vi "FromRepo.vi"(8 "error in":errorcluster, 9 "from repo cluster":T2, 10 "repository in":refnum<class "NISE_CEF_Repository.lvclass">, 11 "engine in":refnum<class "Engine Parent Editor Node.lvclass">) -> (0 "error out":errorcluster, 2 "repository out":refnum<class "NISE_CEF_Repository.lvclass">, 3 "node":T1)   [LabVIEW 2013, in "PL Framework Configuration Tool.lvlib" / "Engine Parent Editor Node.lvclass"]
doc: "Grabs information from the Repo and stores it in the nodes."
uses:
  Engine Parent Editor Node.lvclass
  <vilib>/CEF_TreeControl/Repository/NISE_CEF_Repository.lvclass
  <vilib>/CEF_TreeControl/Node/FromRepoCluster.ctl
  <vilib>/CEF_TreeControl/Node/NodeRef.ctl
  <vilib>/CEF_TreeControl/Node/NISE_CEF_Node.lvclass
  Framework Configuration Classes/platypus configuration/engines cluster.ctl
  <vilib>/NI/Module Execution Interface/Engine Configuration/engine configuration.lvclass
  <vilib>/NI/Tag Bus Module Framework/module configuration/TBM module configuration.lvclass
  EngineTags/EngineTags.lvclass
  Engine Mappings/Engine Mappings.lvclass
  TBM Configuration Node/TBM Configuration Node.lvclass
  <vilib>/NI/Tag Bus Module Framework/root configuration/TBM configuration.lvclass/TBM configuration.ctl
  Framework Configuration Classes/class cache/class type.ctl
  <vilib>/NI/Tag Bus Module Framework/root configuration/create GUID.vi
  <vilib>/NI/Tag Bus Module Framework/root configuration/read metadata property.vi
  Framework Configuration Classes/class cache/PL_class cache.lvlib
  Framework Configuration Classes/platypus configuration/PLConfigurationSerializer.lvlib
  <vilib>/NI/Tag Bus Module Framework/root configuration/TBM configuration.lvclass
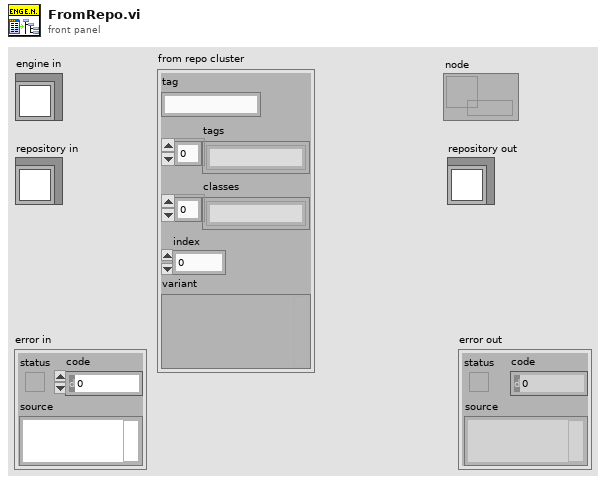
[diagram p1: front panel]
types:
  T1 = typedef "NISE_CEF_Node.lvclass/NodeRef.ctl" = refnum<data-value>
  T2 = typedef "NISE_CEF_Node.lvclass/FromRepoCluster.ctl" = cluster{"tag":string, "tags":string[], "classes":string[], "index":i32, "variant":variant}
  T3 = typedef "PLConfigurationSerializer.lvlib/engines cluster.ctl" = cluster{"engine configuration":refnum<class "engine configuration.lvclass">, "modules":refnum<class "TBM module configuration.lvclass">[]}
  T4 = typedef "PL_class cache.lvlib/class type.ctl" = enum16{"unused", "other pl", "system", "target", "engine", "module"}
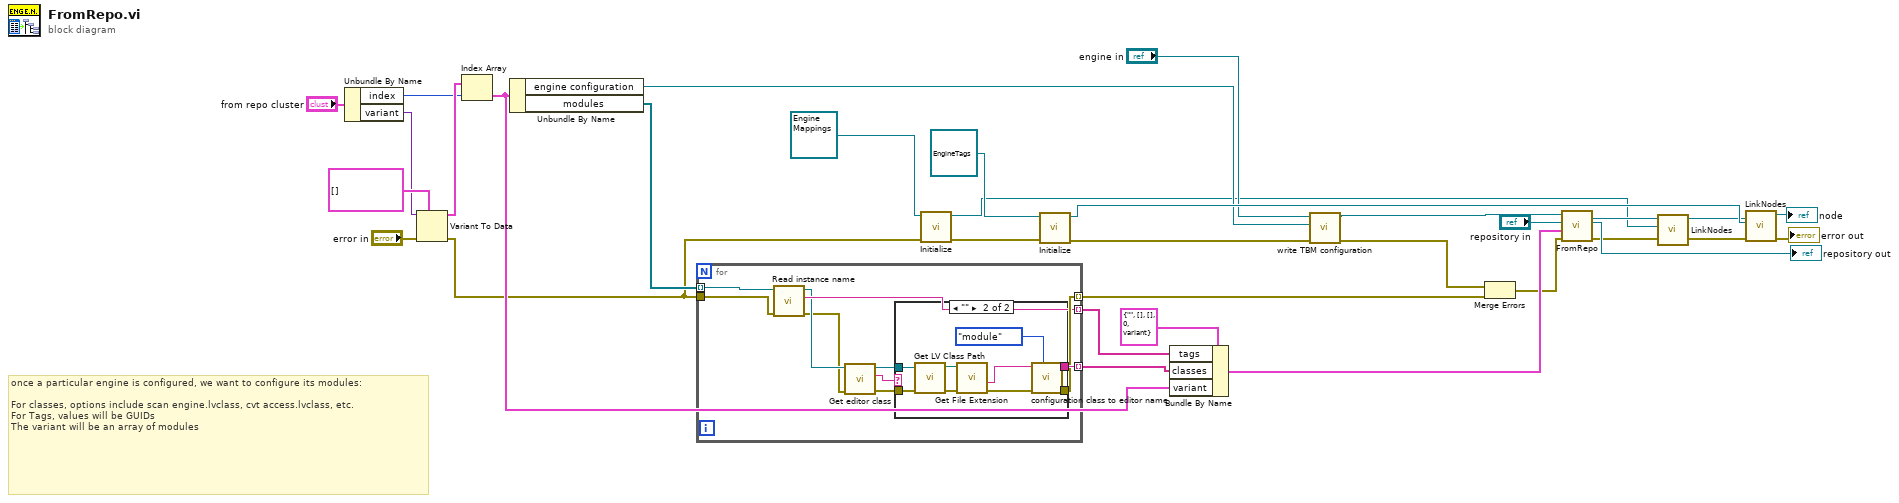
[diagram p0: block diagram]
diagram:
  # "once a particular engine is configured, we want to configure its modules:\n\nFor classes, options include scan engine.lvclass, cvt access.lvclass, etc.\nFor Tags, values will be GUIDs\nThe variant will be an array of modules"
  n1 = Unbundle By Name("from repo cluster") -> ("index"=w31:i32, "variant"=w30:variant)
  n2 = Variant To Data(error in="error in", type=T3[] [], Variant=w30) -> (data=w32:T3[], error out=w1:errorcluster)
  n3 = Index Array(array=w32, index=w31) -> (element=w14:T3)
  n4 = Unbundle By Name(w14) -> ("engine configuration"=w12:refnum<class "engine configuration.lvclass">, "modules"=w15:refnum<class "TBM module configuration.lvclass">[])
  n5 = for {
    tunnel: w15 -> [w43] mode=indexing
    tunnel: [w39] -> w28 mode=indexing
    tunnel: [w42] -> w27 mode=indexing
    tunnel: w1 -> [w40]
    tunnel: [w41] -> w18 mode=indexing
    n6 = call <vilib>:"Read instance name.vi"("error in"=w40, "configuration in"=w43) -> ("error out"=w37:errorcluster, "instance id"=w39:string, "configuration out"=w38:refnum<class "TBM module configuration.lvclass">)  [unwired: 7 in]
    n7 = call "Get editor class.vi"("error in"=w37, "configuration in"=w38) -> ("error out"=w35:errorcluster, "editor class"=w34:string, "configuration out"=w36:refnum<class "TBM module configuration.lvclass">)  [unwired: 7 in]
    n8 = case shown="\"\"" w34 {
      selector: w34 -> [w44 _]
      tunnel: [w44 w54] -> w42
      tunnel: [w45 w52] -> w41
      tunnel: w36 -> [_ w50]
      tunnel: w35 -> [w45 w46]
      frame Default {
      }
      frame "" {
        n9 = call <vilib>:"Get LV Class Path.vi"("error in (no error)"=w46, "object"=w50) -> ("error out"=w51:errorcluster, "class path"=w49:path)  [unwired: 8 in]
        n10 = call <vilib>:"Get File Extension.vi"("error in (no error)"=w51, "file"=w49) -> ("error out"=w47:errorcluster, "filename without extension"=w48:string)  [unwired: 6 in, 2 out]
        n11 = call "configuration class to editor name.vi"("class type"=class_type."module", "error in"=w47, "configuration class name"=w48) -> ("error out"=w52:errorcluster, "editor node class name"=w54:string)  [unwired: 7 in]
      }
    }
  }
  n12 = call-dynamic "Initialize.vi"("error in"=w1, "node in"=refnum<class "Engine Mappings.lvclass"> refnum ("PL Framework Configuration Tool.lvlib:Engine Mapping Viewer")) -> ("error out"=w4:errorcluster, "data value reference"=w2:T1)  [unwired: 7 in, 1 out]
  n13 = call-dynamic "Initialize.vi"("error in"=w4, "node in"=refnum<class "EngineTags.lvclass"> refnum ("EngineTags.lvclass")) -> ("error out"=w11:errorcluster, "data value reference"=w26:T1)  [unwired: 7 in, 1 out]
  n14 = Bundle By Name(cluster=T2 {"tag"="", "tags"=[], "classes"=[], "index"=0, "variant"=variant} ("from repo cluster"), "tags"=w28, "classes"=w27, "variant"=w14) -> (w25:T2)
  n15 = call-dynamic "write TBM configuration.vi"("error in"=w11, "configuration"=w12, "TBM Configuration Node in"="engine in") -> ("error out"=w10:errorcluster, "TBM Configuration Node out"=w9:refnum<class "Engine Parent Editor Node.lvclass">)  [unwired: 7 in]
  n16 = Merge Errors(w10, w18) -> (w17:errorcluster)
  n17 = call-parent "FromRepo.vi"("error in"=w17, "from repo cluster"=w25, "repository in"="repository in", "node in"=w9) -> ("error out"=w8:errorcluster, "repository out"=→"repository out":refnum<class "NISE_CEF_Repository.lvclass">, "node"=w7:T1)  [unwired: 5 in]
  n18 = call <vilib>:"LinkNodes.vi"("error in"=w8, "child in"=w2, "parent in"=w7) -> ("error out"=w5:errorcluster, "parent out"=w6:T1)  [unwired: 6 in, 1 out]
  n19 = call <vilib>:"LinkNodes.vi"("error in"=w5, "child in"=w26, "parent in"=w6) -> ("error out"=→"error out":errorcluster, "parent out"=→"node":T1)  [unwired: 6 in, 1 out]
